vi "State-Phi.vi"(8 "error in (no error)":errorcluster, 9 "Inner Loop State in":T2 {"Theta (Deg)" format="%#_3g"; "Theta (Rad)" format="%#_3g"; "eTheta" format="%#_3g"; "Steering U" format="%#_2g"}, 10 "Gamma Setpoint":dbl, 11 "Phi Setpoint":dbl) -> (0 "error out":errorcluster, 1 "Outer Loop State out":T1 {"Phi Setpoint" format="%#_13g"})   [LabVIEW 2014]
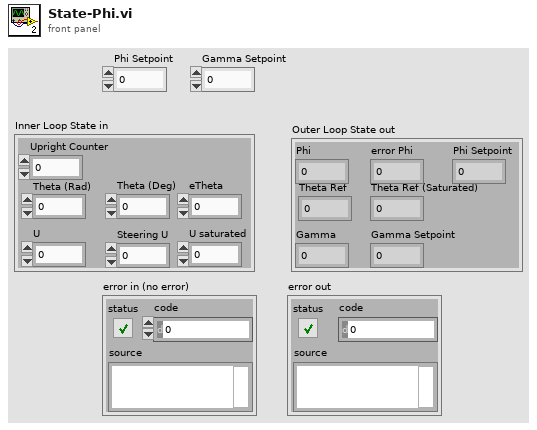
[diagram p1: front panel]
types:
  T1 = cluster{"Phi":dbl, "error Phi":dbl, "Gamma":dbl, "Theta Ref":dbl, "Theta Ref (Saturated)":sgl, "Gamma Setpoint":dbl, "Phi Setpoint":dbl}
  T2 = cluster{"Upright Counter":dbl, "Theta (Deg)":dbl, "Theta (Rad)":dbl, "eTheta":dbl, "U":dbl, "Steering U":dbl, "U saturated":sgl}
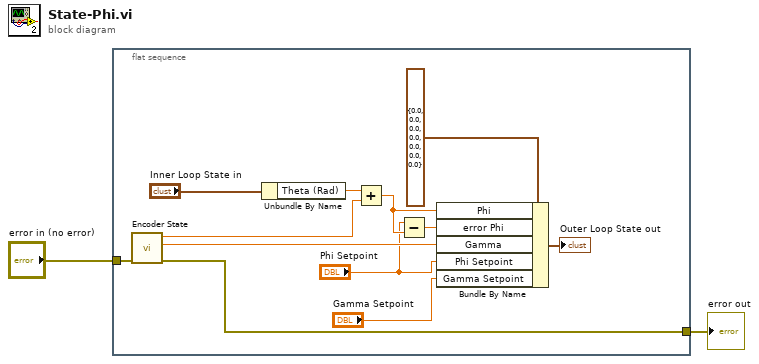
[diagram p0: block diagram]
diagram:
  n1 = flat-sequence {
    tunnel: "error in (no error)" -> [w14]
    tunnel: [w13] -> w1
    frame #0 {
      n2 = call "Encoder State.vi"("error in (no error)"=w14) -> ("error out"=w13:errorcluster, "Gamma"=w7:dbl, "Combined Wheel Angle"=w8:dbl)  [unwired: 8 in]
      n3 = Unbundle By Name("Inner Loop State in") -> ("Theta (Rad)"=w11:dbl)
      n4 = Add(x=w11, y=w8) -> (x+y=w10:dbl)
      n5 = Subtract(x="Phi Setpoint", y=w10) -> (x-y=w9:dbl)
      n6 = Bundle By Name(cluster=T1 {"Phi"=0.0, "error Phi"=0.0, "Gamma"=0.0, "Theta Ref"=0.0, "Theta Ref (Saturated)"=0.0, "Gamma Setpoint"=0.0, "Phi Setpoint"=0.0} ("Outer Loop State"), "Phi"=w10, "error Phi"=w9, "Gamma"=w7, "Phi Setpoint"="Phi Setpoint", "Gamma Setpoint"="Gamma Setpoint") -> (→"Outer Loop State out":T1)
    }
  }
  "error out" <- w1
